vi "Conversion.vi"(0 "RowNum":i32, 1 "Y":dbl[](array[numeric]), 2 "ComlNum":i32, 3 "X":dbl[](array[numeric]), 4 "Z":dbl[](array[numeric])) -> (5 "YVector":dbl[](array[numeric]), 6 "XVector":dbl[](array[numeric]), 7 "ZMatrix":T1)   [LabVIEW 2014]
uses:
  <vilib>/Analysis/Matrix/Datatypes/RealMatrix.ctl
  <vilib>/Analysis/Matrix/Numeric/Conversions/Array To Matrix - RA2.vi
  <vilib>/Analysis/Matrix/NI_Matrix.lvlib
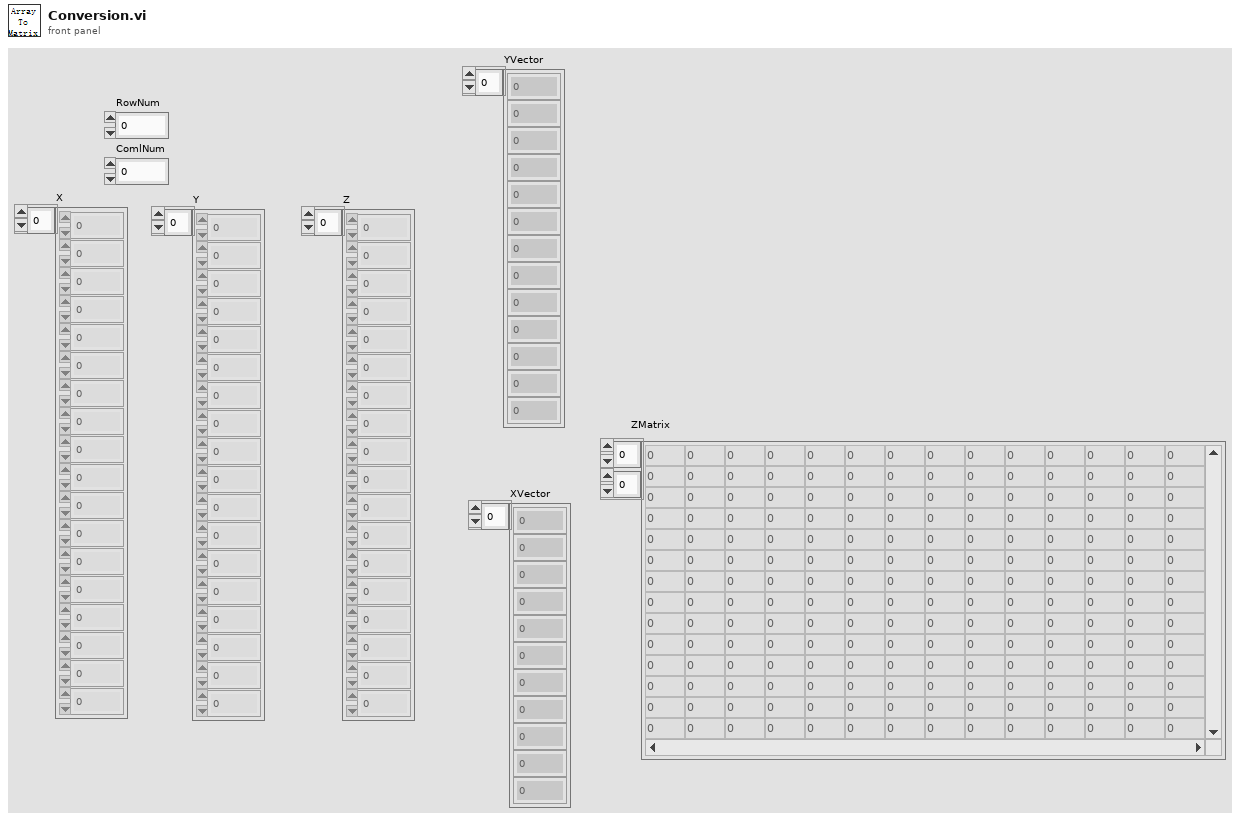
[diagram p1: front panel]
types:
  T1 = typedef "NI_Matrix.lvlib/RealMatrix.ctl" = dbl[][]
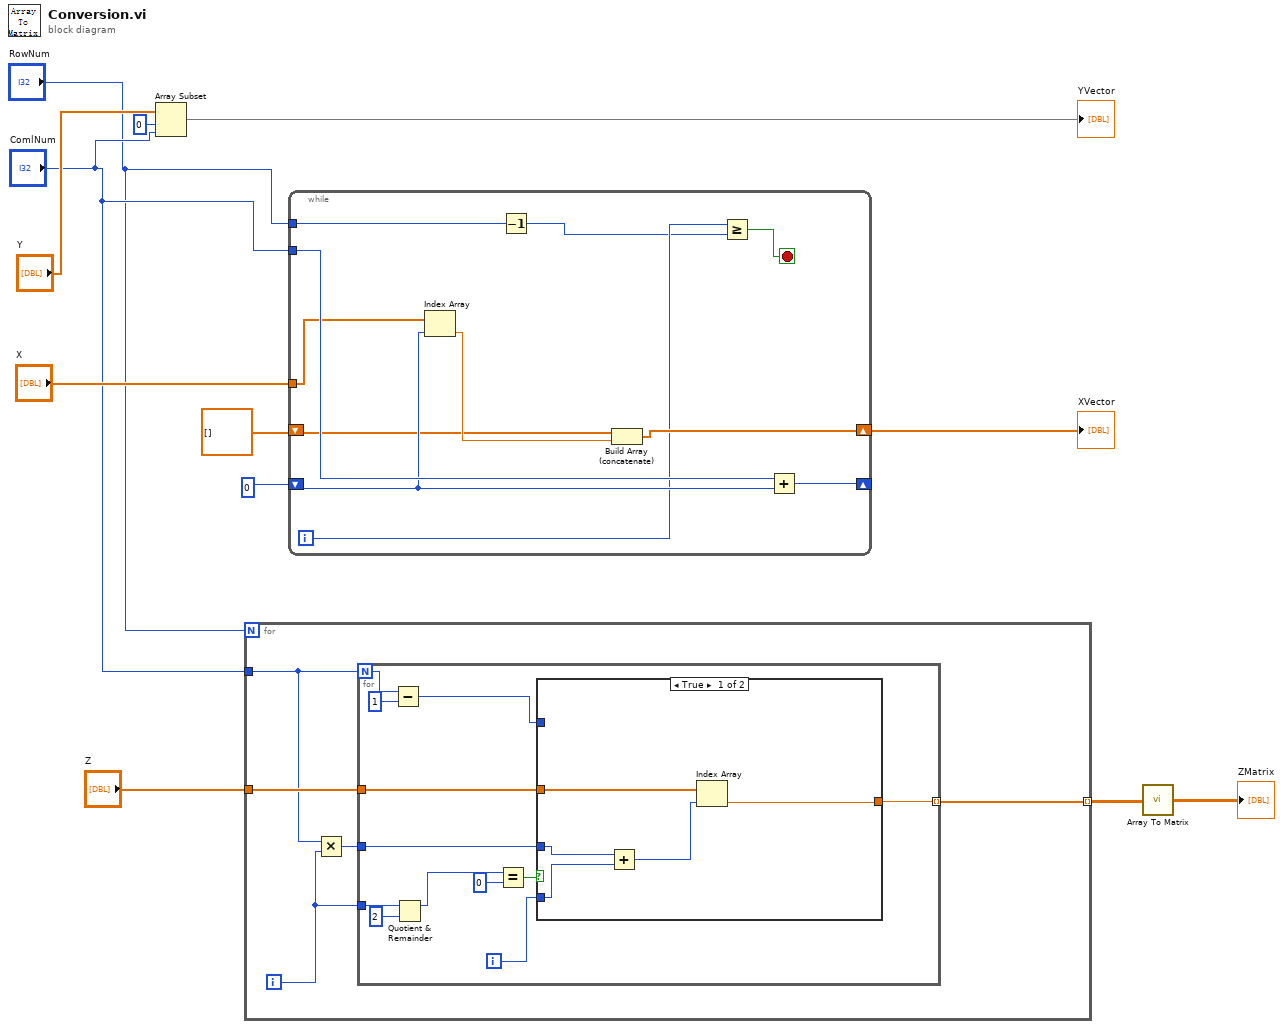
[diagram p0: block diagram]
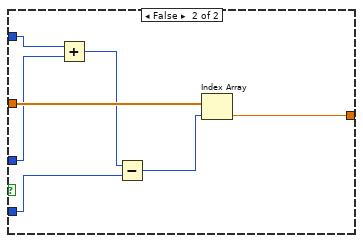
[diagram p2: hidden frame]
diagram:
  n1 = Array Subset(array="Y", index=0, length="ComlNum") -> (→"YVector":dbl[])
  n2 = for {
    N: "RowNum" -> [_]
    tunnel: "ComlNum" -> [w16]
    tunnel: "Z" -> [w17]
    tunnel: [w13] -> w6 mode=indexing
    i -> [w14]
    n3 = Multiply(x=w16, y=w14) -> (x*y=w15:i32)
    n4 = for {
      N: w16 -> [w22]
      tunnel: w17 -> [w29]
      tunnel: w15 -> [w19]
      tunnel: [w28] -> w13 mode=indexing
      tunnel: w14 -> [w27]
      i -> [w18]
      n5 = Subtract(x=w22, y=1) -> (x-y=w20:i32)
      n6 = Quotient & Remainder(x=w27, y=2) -> (x-y*floor(x/y)=w24:i32)  [unwired: 1 out]
      n7 = Equal?(x=w24, y=0) -> (x = y?=w25:bool)
      n8 = case shown="True" w25 {
        tunnel: w29 -> [w34 w41]
        tunnel: [w33 w40] -> w28
        tunnel: w20 -> [_ w39]
        tunnel: w19 -> [w32 w38]
        tunnel: w18 -> [w31 w37]
        frame True {
          n9 = Add(x=w32, y=w31) -> (x+y=w30:i32)
          n10 = Index Array(array=w34, index=w30) -> (element=w33:dbl)
        }
        frame False {
          n11 = Add(x=w39, y=w38) -> (x+y=w36:i32)
          n12 = Subtract(x=w36, y=w37) -> (x-y=w35:i32)
          n13 = Index Array(array=w41, index=w35) -> (element=w40:dbl)
        }
      }
    }
  }
  n14 = while {
    tunnel: "ComlNum" -> [w51]
    tunnel: "X" -> [w50]
    shift-right: [w52] -> _
    shift-left: 0 -> [w49]
    shift-right: [w46] -> w2
    shift-left: dbl[] [] -> [w47]
    tunnel: "RowNum" -> [w43]
    i -> [w44]
    stop <- w45 stop-if-true
    n15 = Index Array(array=w50, index=w49) -> (element=w48:dbl)
    n16 = Decrement(x=w43) -> (x-1=w42:i32)
    n17 = Build Array (concatenate)(w47, w48) -> (w46:dbl[])
    n18 = Greater Or Equal?(x=w44, y=w42) -> (x >= y?=w45:bool)
    n19 = Add(x=w51, y=w49) -> (x+y=w52:i32)
  }
  "XVector" <- w2
  n20 = call-poly <vilib>:"Array To Matrix.vi"("Real 2D Array"=w6) -> ("Real Matrix"=→"ZMatrix":T1)
